vi "Get_Array_of_Channel_Names.vi"() -> ()   [LabVIEW 2014]
uses:
  Sub VIs/ADAM Controls/Channel_names.ctl
panel:
  out "Sub set":string[](array[string])
  in  "length":i32
  in  "Start index":i32
  out "All Active Ch names":string[](array[string])
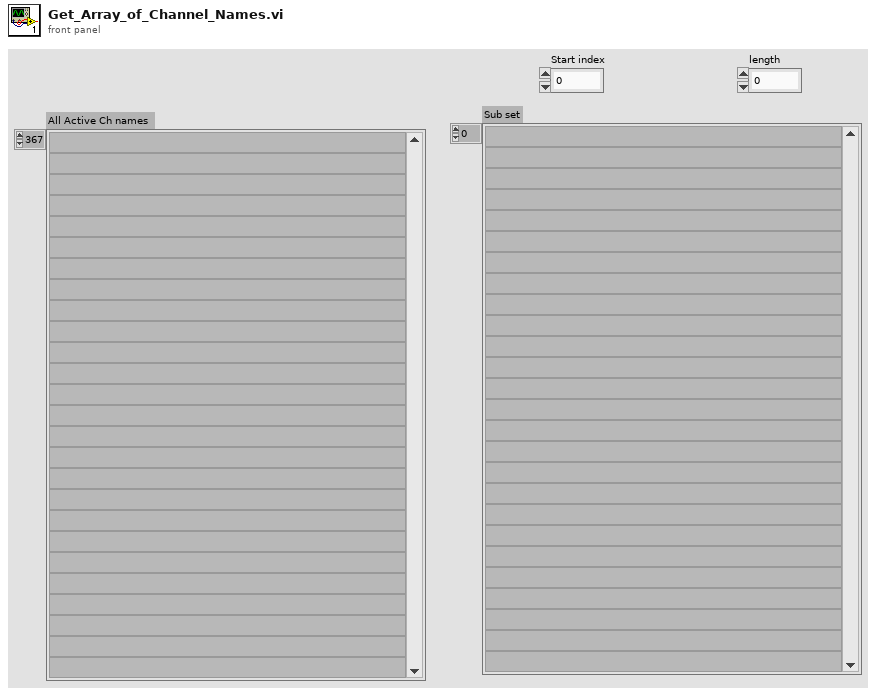
[diagram p1: front panel]
types:
  T1 = typedef "Channel_names.ctl" = enum16{"Active Only", "Active + Off", "All Channels"}
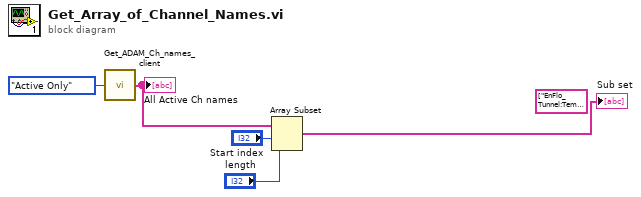
[diagram p0: block diagram]
diagram:
  (unwired) string[] ["EnFlo_Tunnel:Temp_Rake_Y+ve:Z=50", "EnFlo_Tunnel:Temp_Rake_Y+ve:Z=100", "EnFlo_Tunnel:Temp_Rake_Y+ve:Z=150", "EnFlo_Tunnel:Temp_Rake_Y+ve:Z=200", "EnFlo_Tunnel:Temp_Rake_Y+ve:Z=250", "EnFlo_Tunnel:Temp_Rake_Y+ve:Z=300", "EnFlo_Tunnel:Temp_Rake_Y+ve:Z=400", "EnFlo_Tunnel:Temp_Rake_Y+ve:Z=500", "EnFlo_Tunnel:Temp_Rake_Y+ve:Z=600", "EnFlo_Tunnel:Temp_Rake_Y+ve:Z=700", "EnFlo_Tunnel:Temp_Rake_Y+ve:Z=800", "EnFlo_Tunnel:Temp_Rake_Y+ve:Z=900", "EnFlo_Tunnel:Temp_Rake_Y+ve:Z=1000", "EnFlo_Tunnel:Temp_Rake_Y+ve:Z=1100", "EnFlo_Tunnel:Temp_Rake_Y+ve:Z=1225", "EnFlo_Tunnel:Temp_Rake_Y+ve:Z=1350"] ("Sub set")
  n1 = call "Get_ADAM_Ch_names_client.vi"("Channel names set"=Channel_names."Active Only") -> ("Ch names"=w2:string[])
  "All Active Ch names" <- w2
  n2 = Array Subset(array=w2, index="Start index", length="length") -> (→"Sub set":string[])
